vi "Disconnect FlexLogger.vi"(6 "timeout (ms)":i32=-1, 8 "error in (no error)":errorcluster, 11 "FlexLogger_gRPCAPI in":refnum<class "FlexLogger_gRPC.lvclass">) -> (0 "error out":errorcluster, 3 "FlexLogger_gRPCAPI out":refnum<class "FlexLogger_gRPC.lvclass">)   [LabVIEW 2020, in "FlexLogger_gRPC.lvlib" / "FlexLogger_gRPC.lvclass"]
uses:
  FlexLogger_gRPC.lvclass
  FlexLogger_gRPC.lvclass/FlexLogger_gRPC.ctl
  FlexLogger_client/FlexLogger_client.lvlib
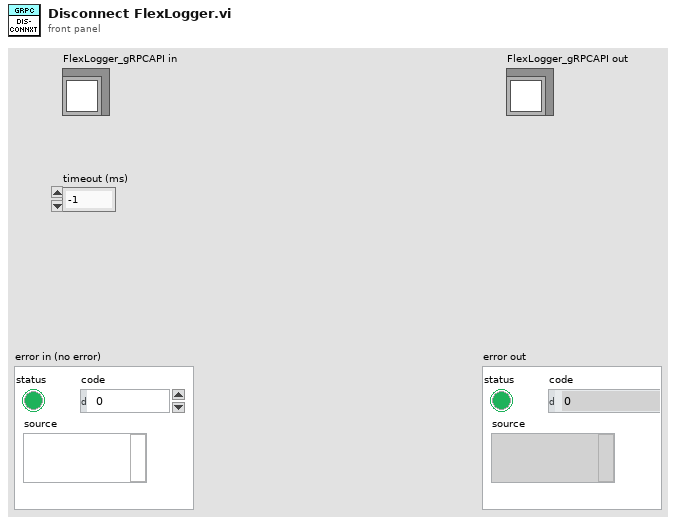
[diagram p1: front panel]
types:
  T1 = typedef "grpc-lvsupport-release.lvlib/grpcId.ctl" = u64
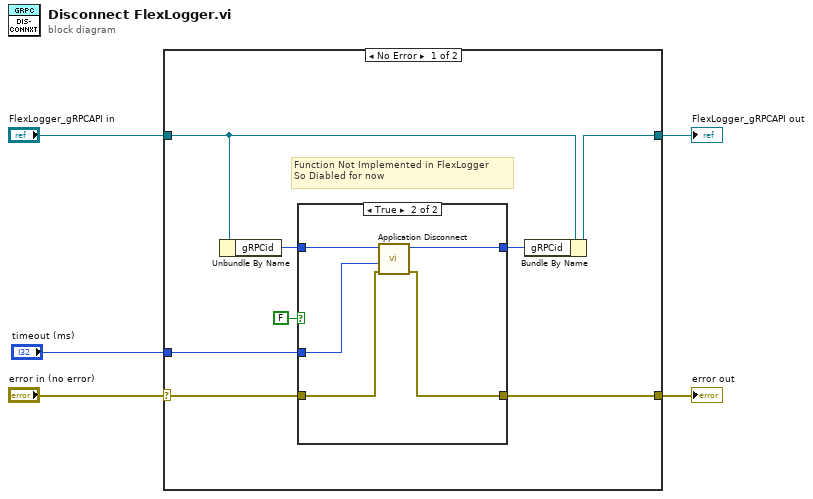
[diagram p0: block diagram]
diagram:
  n1 = case shown="No Error" "error in (no error)" {
    selector: "error in (no error)" -> [w9 w21]
    tunnel: [w8 w21] -> w4
    tunnel: [w12 w22] -> w3
    tunnel: "FlexLogger_gRPCAPI in" -> [w11 w22]
    tunnel: "timeout (ms)" -> [w6 _]
    frame No Error {
      # "Function Not Implemented in FlexLogger\nSo Diabled for now"
      n2 = Unbundle By Name(w11) -> ("gRPCid"=w10:T1)
      n3 = case shown="True" FALSE {
        tunnel: [w15 w20] -> w13
        tunnel: w10 -> [w15 w19]
        tunnel: w9 -> [w14 w18]
        tunnel: [w14 w17] -> w8
        tunnel: w6 -> [_ w16]
        frame False {
        }
        frame True {
          n4 = call "Application Disconnect.vi"("error in"=w18, "timeout (ms)"=w16, "gRPC ID"=w19) -> ("error out"=w17:errorcluster, "gRPC ID out"=w20:T1)  [unwired: 6 in, 1 out]
        }
      }
      n5 = Bundle By Name(cluster=w11, "gRPCid"=w13) -> (w12:refnum<class "FlexLogger_gRPC.lvclass">)
    }
    frame Error {
    }
  }
  "error out" <- w4
  "FlexLogger_gRPCAPI out" <- w3
